vi "Match VI Window With TabControl.vi"(10 "TabCtl Reference":refnum<vi>, 11 "VI Reference":refnum<vi>) -> ()   [LabVIEW 2020]
uses:
  <vilib>/Utility/miscctls.llb/LVPositionTypeDef.ctl
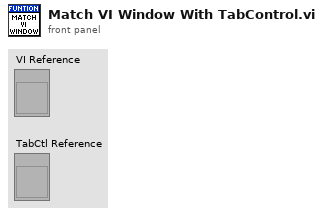
[diagram p1: front panel]
types:
  T1 = typedef "LVPositionTypeDef.ctl" = cluster{"Left":i32, "Top":i32}
  T2 = typedef "LVRectTypeDef.ctl" = cluster{"Left":i16, "Top":i16, "Right":i16, "Bottom":i16}
  T3 = typedef "LVBoundsTypeDef.ctl" = cluster{"Width":u32, "Height":u32}
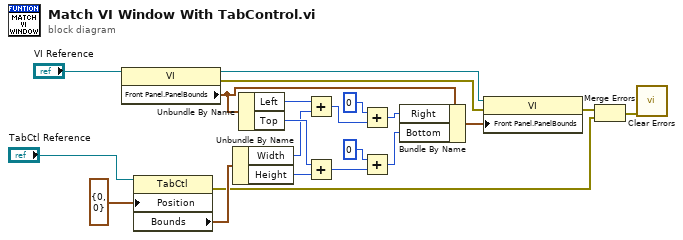
[diagram p0: block diagram]
diagram:
  n1 = property class="VI"(reference="VI Reference") -> (reference out=w12:refnum<vi>, error out=w3:errorcluster, "Front Panel.PanelBounds"=w13:T2)  [unwired: 1 in]
  n2 = property class="TabCtl"(reference="TabCtl Reference", "Position"=T1 {"Left"=0, "Top"=0} ("位置")) -> (error out=w4:errorcluster, "Bounds"=w15:T3)  [unwired: 1 in, 1 out]
  n3 = Unbundle By Name(w15) -> ("Width"=w16:u32, "Height"=w19:u32)
  n4 = Unbundle By Name(w13) -> ("Left"=w14:i16, "Top"=w18:i16)
  n5 = Add(x=w14, y=w16) -> (x+y=w17:u32)
  n6 = Add(x=w18, y=w19) -> (x+y=w20:u32)
  n7 = Add(x=u32 0, y=w17) -> (x+y=w10:u32)
  n8 = Add(x=u32 0, y=w20) -> (x+y=w8:u32)
  n9 = Bundle By Name(cluster=w13, "Right"=w10, "Bottom"=w8) -> (w21:T2)
  n10 = property class="VI"(reference=w12, error in=w3, "Front Panel.PanelBounds"=w21) -> (error out=w5:errorcluster)  [unwired: 1 out]
  n11 = Merge Errors(w5, w4) -> (w2:errorcluster)
  n12 = call <vilib>:"Clear Errors.vi"("error in (no error)"=w2) -> ()  [unwired: 5 in, 2 out]
